vi "Unit_Test_Driver.vi"() -> ()   [LabVIEW 2019]
uses:
  <userlib>/LevyLab/Relay Box/Typedefs/Resistor--enum.ctl
  <userlib>/LevyLab/Relay Box/Relay-Box.lvclass
  lvsrc/subVIs/AFM API/AFM_Driver_Manager/AFM_Driver_Manager.PublicMethods.ctl
  lvsrc/subVIs/AFM API/AFM_Driver_Manager/AFM_Driver_Manager.lvclass
  lvsrc/subVIs/AFM API/AFM_Driver_Manager/AFM_Driver_Manager.PublicEvents.ctl
  <vilib>/addons/_JKI Toolkits/Caraya/classes/Test/Test.lvclass
  <vilib>/addons/_JKI Toolkits/Caraya/classes/Assert/Assert.lvclass
  <vilib>/addons/_JKI Toolkits/Caraya/classes/Assert/Assert True.vi
  <vilib>/addons/_JKI Toolkits/Caraya/classes/Assert/Assert Equal Value_Variant.vi
  <vilib>/addons/_JKI Toolkits/Caraya/classes/Assert/Assert False.vi
panel:
  in  "Levylab_Public_Events_Do_Not_Rename":T1
  in  "Levylab_Public_Methods_Do_Not_Rename":T2
  # "AFM Driver Template"
  # "UNIT TESTS"
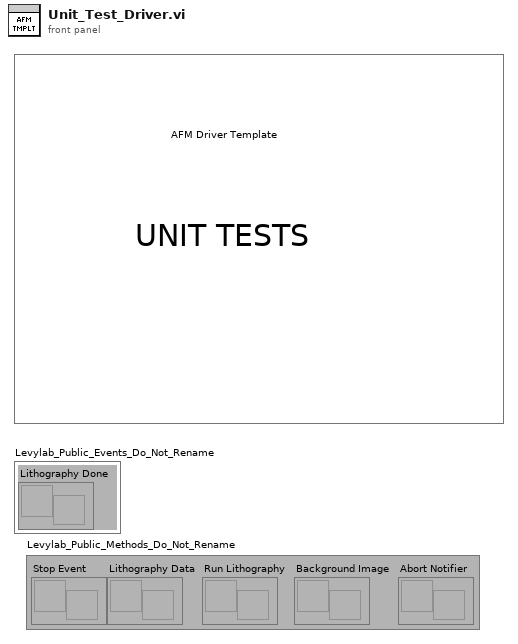
[diagram p1: front panel]
types:
  T1 = typedef "AFM_Driver_Manager.lvclass/AFM_Driver_Manager.PublicEvents.ctl" = cluster{"Lithography Done":refnum<user-event>}
  T2 = typedef "AFM_Driver_Manager.lvclass/AFM_Driver_Manager.PublicMethods.ctl" = cluster{"Stop Event":refnum<user-event>, "Lithography Data":refnum<user-event>, "Run Lithography":refnum<user-event>, "Background Image":refnum<user-event>, "Abort Notifier":refnum<user-event>}
  T3 = typedef "Relay-Box.lvclass/Resistor--enum.ctl" = enum16{"open", "discharge tip", "0 ohms", "100k ohm", "10M ohm", "1G ohm"}
  T4 = cluster{"Name":string, "Litho":cluster{"X":dbl, "Y":dbl, "Speed":dbl, "Voltage":dbl}[], "Set Resistance":T3, "Meta":variant}[]
  T5 = enum32{"Invalid", "Standard", "Closed", "Hidden", "Minimized", "Maximized"}
  T6 = enum32{"invalid app kind", "Development System", "Run Time System", "Student Edition", "Embedded LabVIEW", "Evaluation", "Custom"}
  T7 = cluster{"Core":cluster{"Current VI Reference":refnum<vi>, "Close Panel on Exit?":bool}, "Events":T1, "Lithography Data":cluster{"Name":string, "Litho":cluster{"X":dbl, "Y":dbl, "Speed":dbl, "Voltage":dbl}[], "Set Resistance":T3, "Meta":variant}[], "Background Image":path, "Abort Notifier":refnum<notifier>, "Offsets":cluster{"X":dbl, "Y":dbl}}
  T8 = cluster{"Current VI Reference":refnum<vi>, "Close Panel on Exit?":bool}
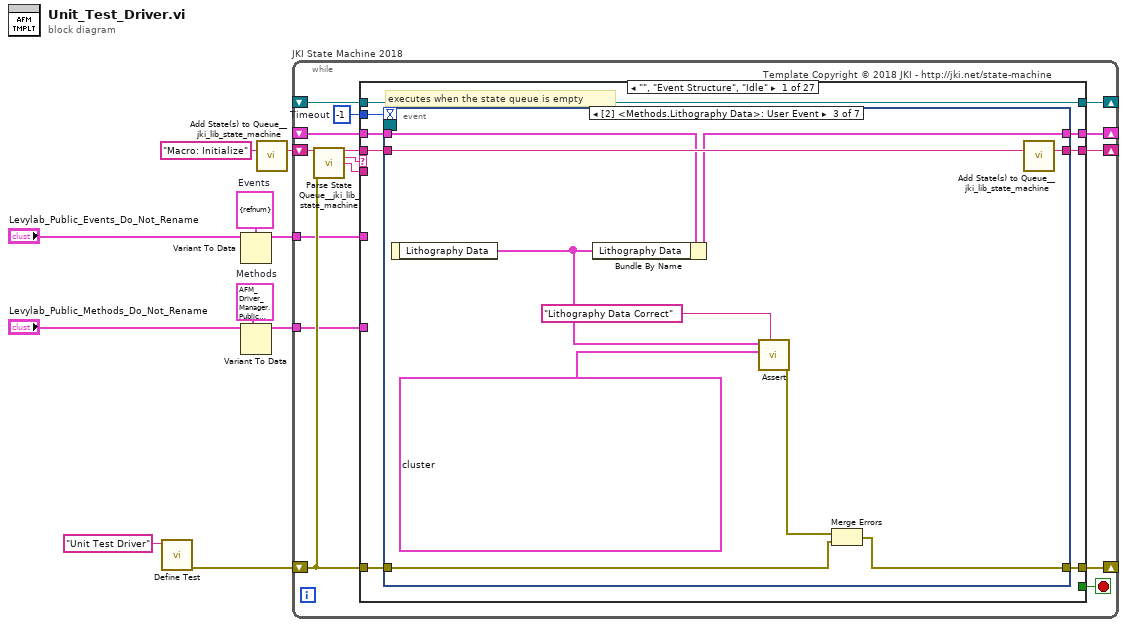
[diagram p0: block diagram]
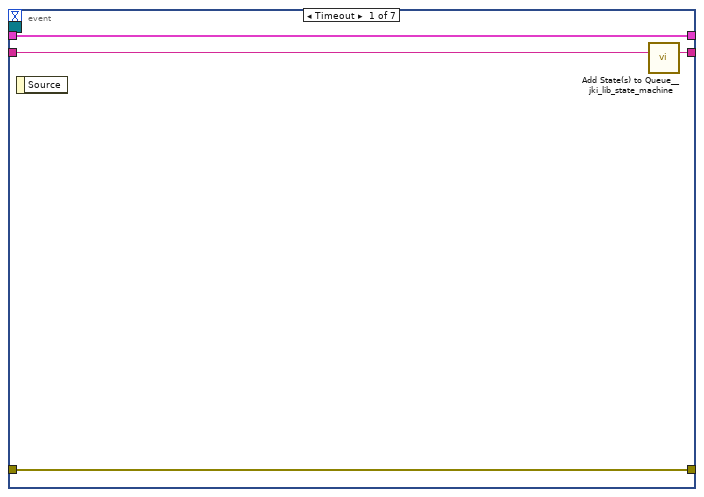
[diagram p2: hidden frame]
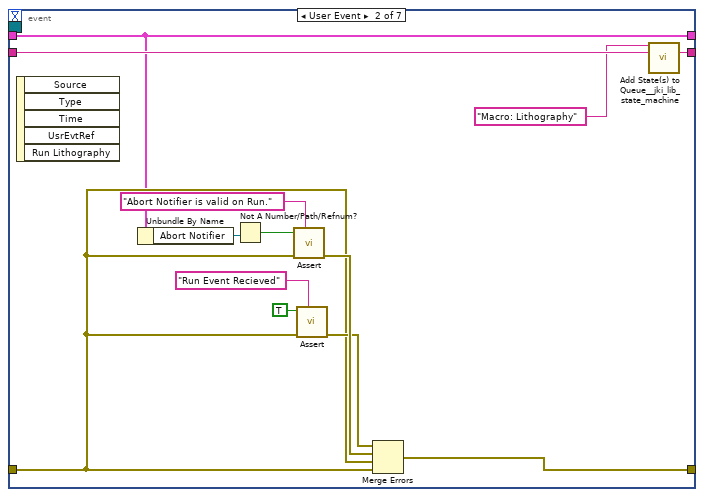
[diagram p3: hidden frame]
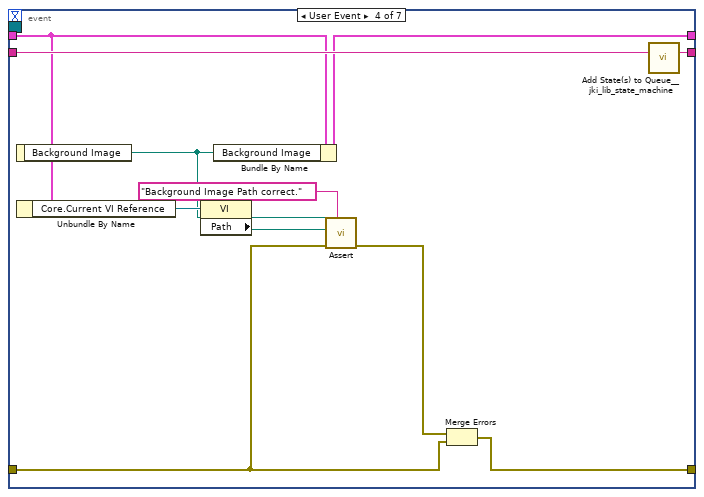
[diagram p4: hidden frame]
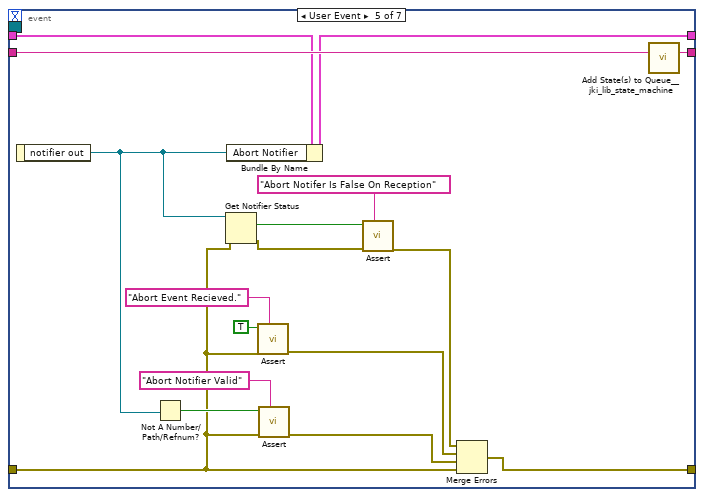
[diagram p5: hidden frame]
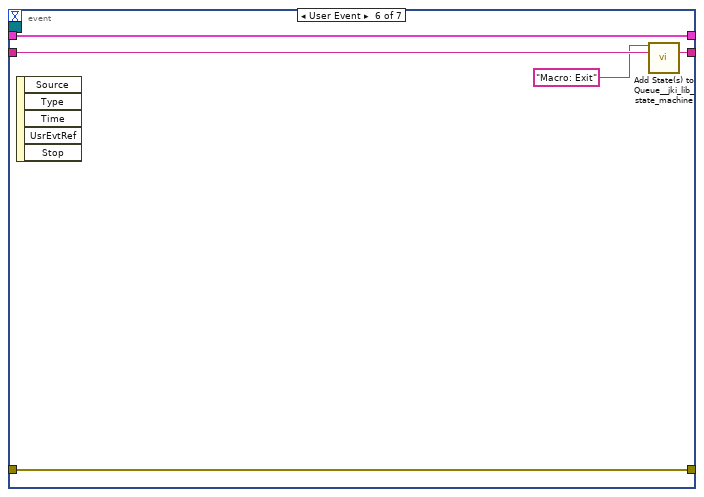
[diagram p6: hidden frame]
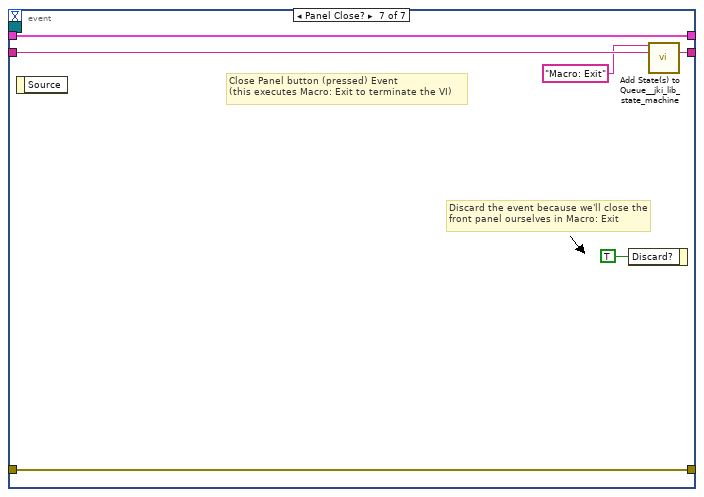
[diagram p7: hidden frame]
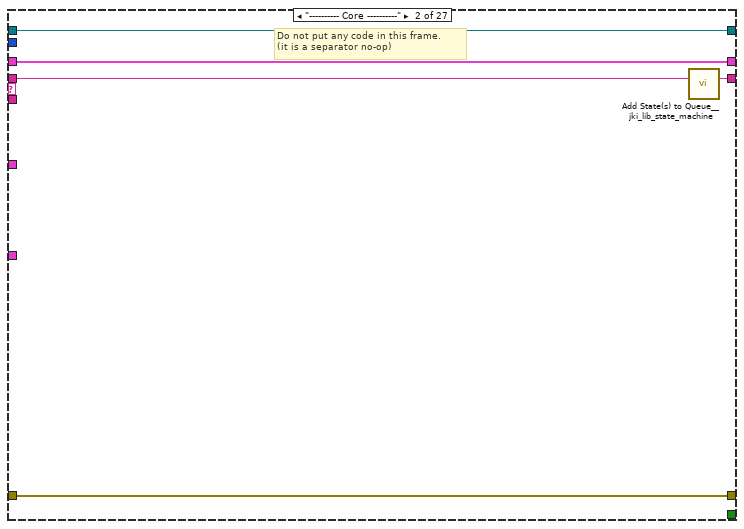
[diagram p8: hidden frame]
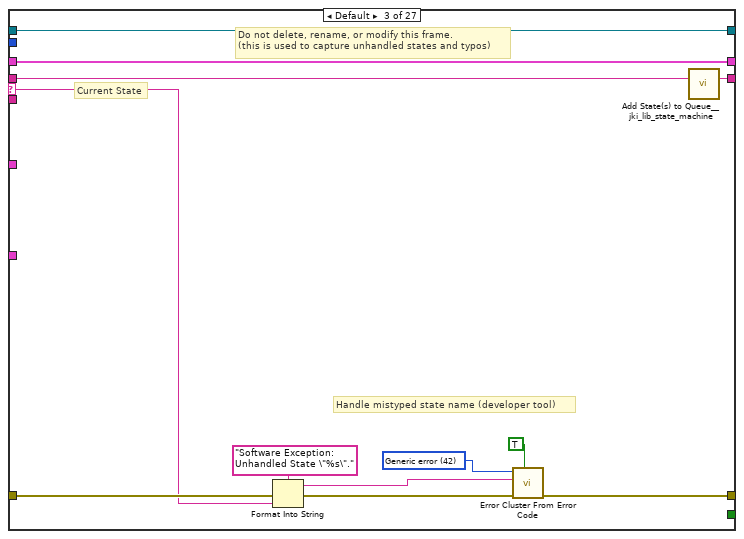
[diagram p9: hidden frame]
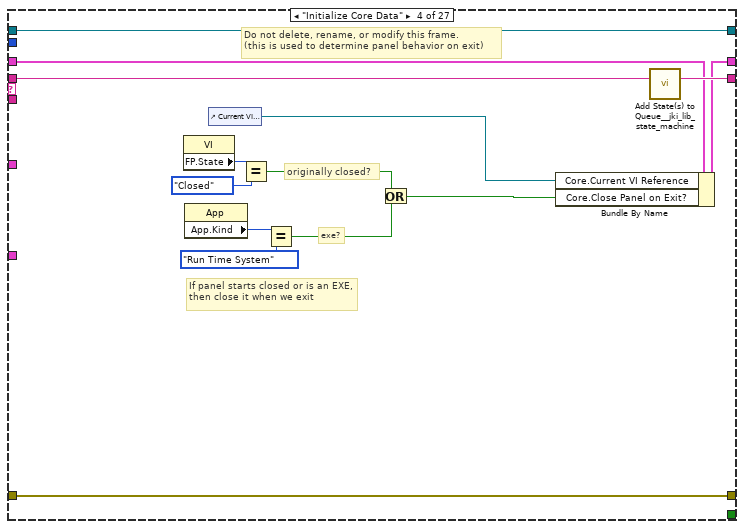
[diagram p10: hidden frame]
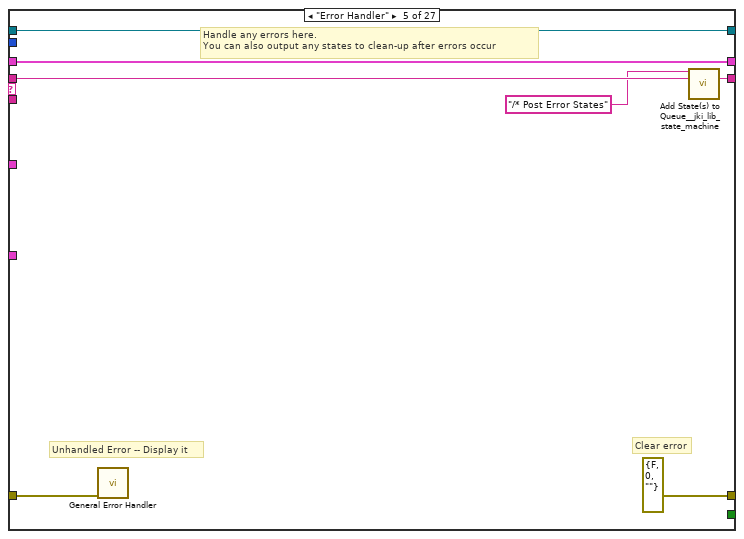
[diagram p11: hidden frame]
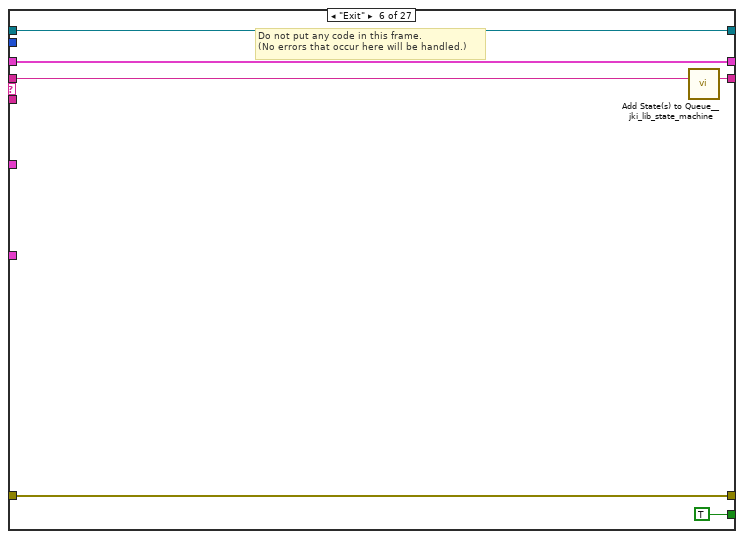
[diagram p12: hidden frame]
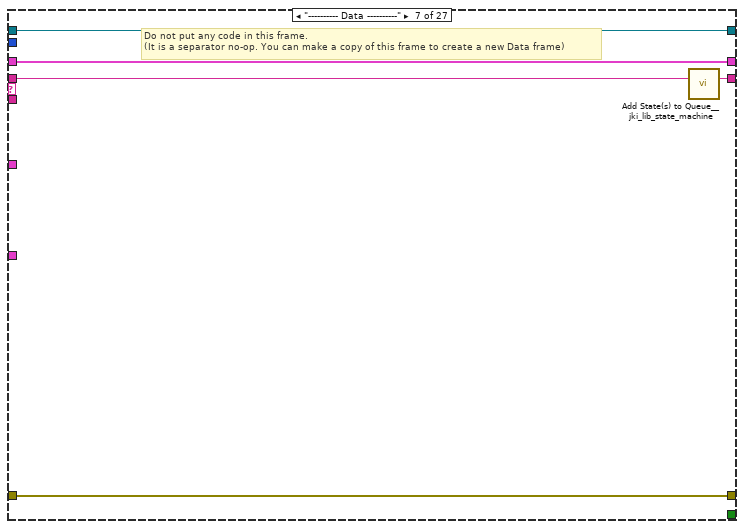
[diagram p13: hidden frame]
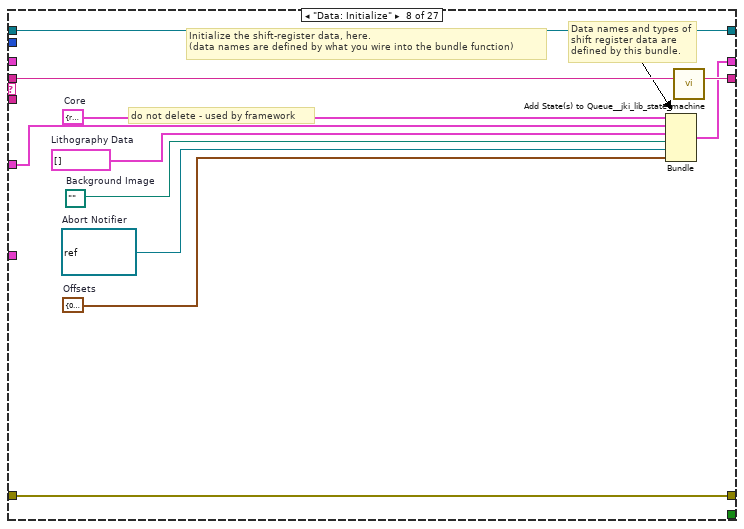
[diagram p14: hidden frame]
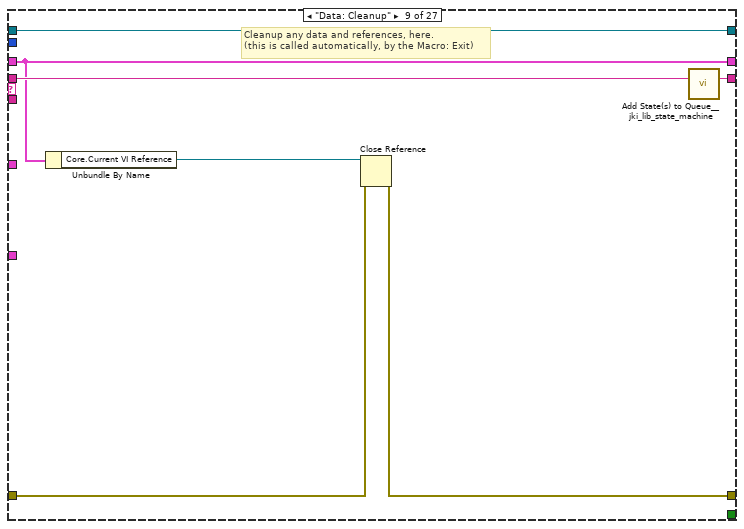
[diagram p15: hidden frame]
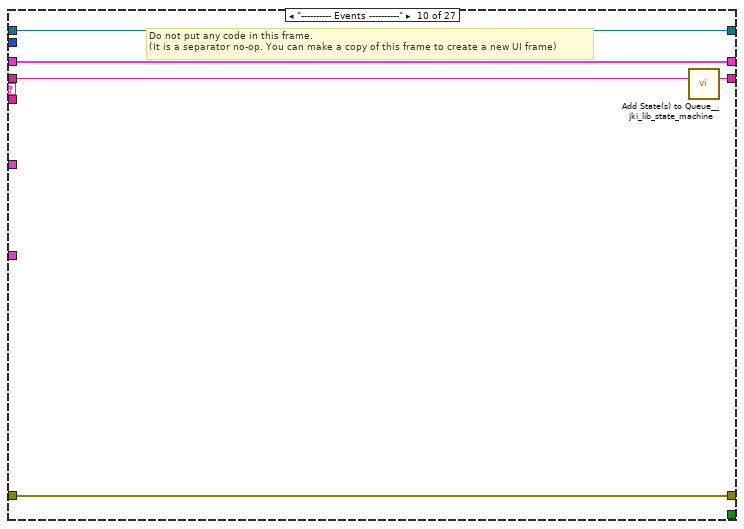
[diagram p16: hidden frame]
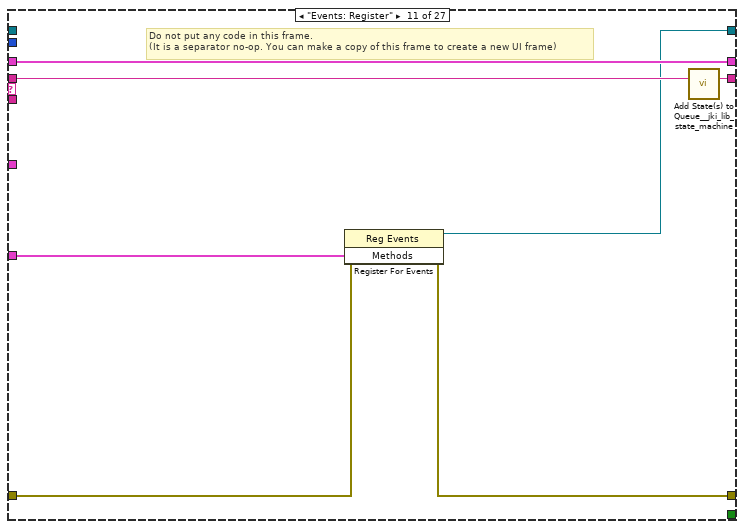
[diagram p17: hidden frame]
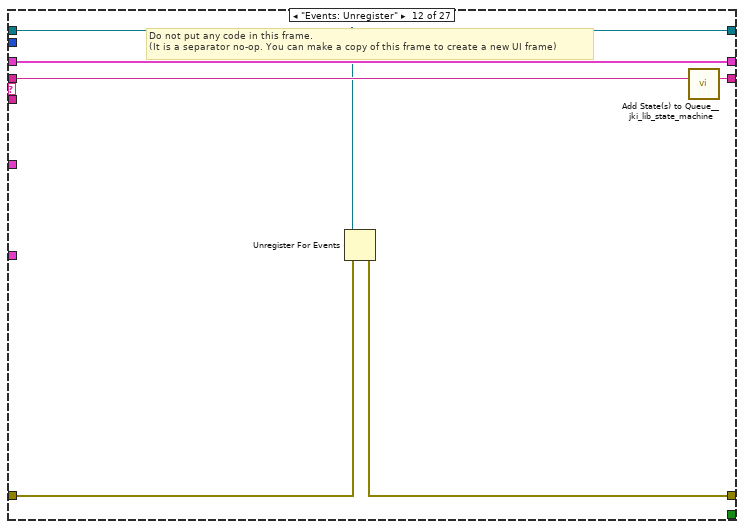
[diagram p18: hidden frame]
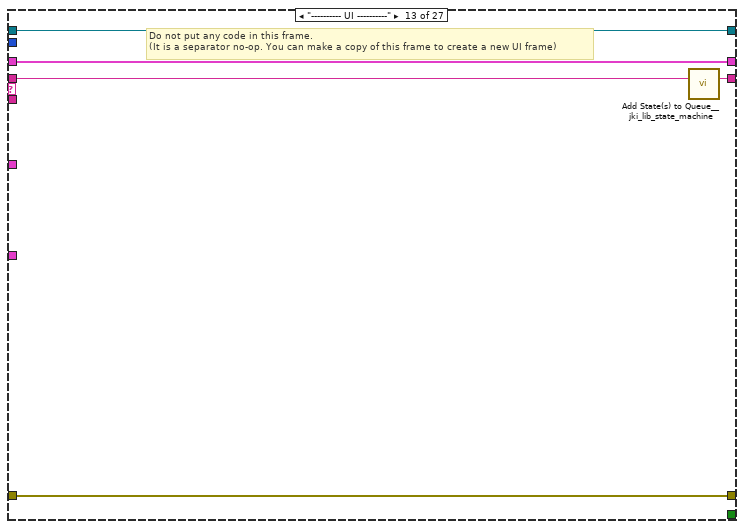
[diagram p19: hidden frame]
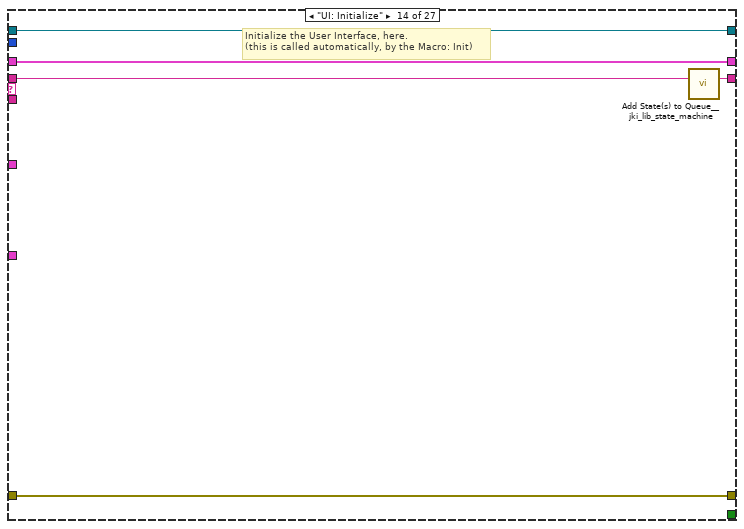
[diagram p20: hidden frame]
diagram:
  w6 = T1 {"Lithography Done"=refnum}  # Events
  w8 = T2 {"Stop Event"=refnum, "Lithography Data"=refnum, "Run Lithography"=refnum, "Background Image"=refnum, "Abort Notifier"=refnum}  # Methods
  n1 = call <vilib>:"Define Test.vi"("Label (VI Title)"="Unit Test Driver") -> ("error out"=w2:errorcluster)  [unwired: 9 in, 1 out]
  n2 = Variant To Data(type=w6, Variant="Levylab_Public_Events_Do_Not_Rename") -> (data=w3:T1)  [unwired: 1 in, 1 out]
  n3 = Variant To Data(type=w8, Variant="Levylab_Public_Methods_Do_Not_Rename") -> (data=w4:T2)  [unwired: 1 in, 1 out]
  n4 = call <vilib>:"Add State(s) to Queue__jki_lib_state_machine.vi"("State(s) in (\"\")"="Macro: Initialize") -> ("States Out"=w10:string)  [unwired: 14 in]
  n5 = while "JKI State Machine 2018" {
    shift-right: [w18] -> _
    shift-left: _ -> [w17]
    shift-right: [w21] -> _
    shift-left: w2 -> [w15]
    shift-right: [w20] -> _
    shift-left: w10 -> [w22]
    tunnel: w4 -> [w11]
    tunnel: w3 -> [w14]
    shift-right: [w13] -> _
    shift-left: _ -> [w12]
    stop <- w19 stop-if-true
    w16 = -1  # Timeout
    # "Template Copyright © 2018 JKI - http://jki.net/state-machine"
    n6 = call <vilib>:"Parse State Queue__jki_lib_state_machine.vi"("State Queue"=w22, "Error In (no error)"=w15) -> ("Remaining States"=w24:string, "Current State"=w25:string, "Arguments"=w23:string)  [unwired: 11 in]
    n7 = case shown="\"\", \"Event Structure\", \"Idle\"" w25 {
      selector: w25 -> [_ _ w106 _ _ _ _ _ _ _ _ _ _ _ _ _ _ _ _ _ _ _ _ _ _ _ _]
      tunnel: w24 -> [w33 w104 w110 w130 w137 w143 w148 w159 w166 w171 w178 w184 w189 w194 w201 w213 w283 w289 w295 w306 w311 w316 w321 w326 w331 w342 w358]
      tunnel: w23 -> [_ _ _ _ _ _ _ _ _ _ _ _ _ _ w196 w207 _ _ _ _ _ _ _ _ _ _ _]
      tunnel: w17 -> [w31 w101 w108 w123 w134 w141 w145 _ w161 w168 w176 w182 w186 w192 w199 w209 w280 w286 w292 w303 w308 w313 w318 w323 w328 w339 w355]
      tunnel: [w30 w102 w112 w127 errorcluster {"status"=FALSE, "code"=0, "source"=""} ("error out") w140 w146 w156 w162 w169 w172 w179 w187 w191 w197 w210 w281 w287 w293 w304 w309 w314 w319 w324 w329 w334 w352] -> w21
      tunnel: w15 -> [w29 w102 w111 w127 w133 w140 w146 w156 w163 w169 w173 w180 w187 w191 w198 w211 w281 w287 w293 w304 w309 w314 w319 w324 w329 w333 w351]
      tunnel: [w32 w103 w109 w129 w136 w142 w147 w158 w165 w170 w177 w183 w188 w193 w200 w212 w282 w288 w294 w305 w310 w315 w320 w325 w330 w341 w357] -> w20
      tunnel: [_ _ _ _ _ TRUE _ _ _ _ _ _ _ _ _ _ _ _ _ _ _ _ _ _ _ _ _] -> w19
      tunnel: [w28 w101 w108 w128 w134 w141 w145 w157 w161 w168 w176 w182 w186 w192 w199 w209 w280 w286 w292 w303 w308 w313 w318 w323 w328 w339 w355] -> w18
      tunnel: w16 -> [w27 _ _ _ _ _ _ _ _ _ _ _ _ _ _ _ _ _ _ _ _ _ _ _ _ _ _]
      tunnel: w14 -> [_ _ _ _ _ _ _ w154 _ _ _ _ _ _ _ _ _ _ _ _ _ _ _ _ _ _ _]
      tunnel: [w26 w100 w105 w117 w131 w138 w144 w150 w160 w167 w175 w181 w185 w190 w195 w206 w279 w284 w291 w296 w307 w312 w317 w322 w327 w340 w356] -> w13
      tunnel: w12 -> [w26 w100 w105 w117 w131 w138 w144 w150 w160 w167 _ w181 w185 w190 w195 w206 w279 w284 w291 w296 w307 w312 w317 w322 w327 w340 w356]
      tunnel: w11 -> [_ _ _ _ _ _ _ _ _ _ w174 _ _ _ _ _ _ _ _ _ _ _ _ _ _ _ _]
      frame "", "Event Structure", "Idle" {
        # "executes when the state queue is empty"
        n8 = event shown="[2] <Methods.Lithography Data>: User Event" {
          selector: w26 -> [_ _ _ _ _ _ _]
          dyn-events: _ -> [_ _ _ _ _ _ _]
          timeout: w27 -> [_ _ _ _ _ _ _]
          tunnel: w33 -> [w37 w50 w60 w71 w88 w93 w99]
          tunnel: [w36 w49 w59 w70 w87 w92 w98] -> w32
          tunnel: w31 -> [w34 w39 w57 w68 w85 w90 w96]
          tunnel: [w35 w43 w53 w63 w80 w91 w97] -> w30
          tunnel: w29 -> [w35 w40 w52 w61 w75 w91 w97]
          tunnel: [w34 w39 w58 w69 w86 w90 w96] -> w28
          event Timeout {
            n9 = event-data() -> ()  [unwired: 1 in, 1 out]
            n10 = call <vilib>:"Add State(s) to Queue__jki_lib_state_machine.vi"("State(s) in (\"\")"=w37) -> ("States Out"=w36:string)  [unwired: 14 in]
          }
          event User Event {
            n11 = event-data() -> ()  [unwired: 1 in, 5 out]
            n12 = Unbundle By Name(w39) -> ("Abort Notifier"=w38:refnum<notifier>)
            n13 = Not A Number/Path/Refnum?(number/path/refnum=w38) -> (NaN/Path/Refnum?=w46:bool)
            n14 = call-poly <vilib>:"Assert.vi"("Label"="Abort Notifier is valid on Run.", "error in (no error)"=w40, "False?"=w46) -> ("error out"=w42:errorcluster)  [unwired: 7 in, 1 out]
            n15 = call-poly <vilib>:"Assert.vi"("Label"="Run Event Recieved", "error in (no error)"=w40, "True?"=TRUE) -> ("error out"=w41:errorcluster)  [unwired: 7 in, 1 out]
            n16 = Merge Errors(w41, w42, w40, w40) -> (w43:errorcluster)
            n17 = call <vilib>:"Add State(s) to Queue__jki_lib_state_machine.vi"("State(s) in Front (\"\")"="Macro: Lithography", "State(s) in (\"\")"=w50) -> ("States Out"=w49:string)  [unwired: 13 in]
          }
          event User Event {
            n18 = event-data() -> ("Lithography Data"=w51:T4)  [unwired: 1 in]
            n19 = Bundle By Name(cluster=w57, "Lithography Data"=w51) -> (w58:T7)
            n20 = call-poly <vilib>:"Assert.vi"("Label"="Lithography Data Correct", "Y"=T4 [{"Name"="p0", "Litho"=[{"X"=1.0, "Y"=2.0, "Speed"=3.0, "Voltage"=4.0}], "Set Resistance"=enum."discharge tip", "Meta"=variant}, {"Name"="p1", "Litho"=[{"X"=5.0, "Y"=6.0, "Speed"=7.0, "Voltage"=8.0}], "Set Resistance"=enum."open", "Meta"=variant}] ("Lithography Data"), "X"=w51) -> ("error out"=w54:errorcluster)  [unwired: 7 in, 1 out]
            n21 = Merge Errors(w54, w52) -> (w53:errorcluster)
            n22 = call <vilib>:"Add State(s) to Queue__jki_lib_state_machine.vi"("State(s) in (\"\")"=w60) -> ("States Out"=w59:string)  [unwired: 14 in]
          }
          event User Event {
            n23 = event-data() -> ("Background Image"=w66:path)  [unwired: 1 in]
            n24 = Unbundle By Name(w68) -> ("Core.Current VI Reference"=w67:refnum<vi>)
            n25 = property class="VI"(reference=w67) -> ("Path"=w65:path)  [unwired: 1 in, 2 out]
            n26 = Bundle By Name(cluster=w68, "Background Image"=w66) -> (w69:T7)
            n27 = call-poly <vilib>:"Assert.vi"("Label"="Background Image Path correct.", "error in (no error)"=w61, "Y"=w65, "X"=w66) -> ("error out"=w62:errorcluster)  [unwired: 6 in, 1 out]
            n28 = Merge Errors(w62, w61) -> (w63:errorcluster)
            n29 = call <vilib>:"Add State(s) to Queue__jki_lib_state_machine.vi"("State(s) in (\"\")"=w71) -> ("States Out"=w70:string)  [unwired: 14 in]
          }
          event User Event {
            n30 = event-data() -> ("notifier out"=w74:refnum<notifier>)  [unwired: 1 in]
            n31 = Not A Number/Path/Refnum?(number/path/refnum=w74) -> (NaN/Path/Refnum?=w82:bool)
            n32 = Get Notifier Status(notifier=w74, error in (no error)=w75) -> (current notification=w73:bool, error out=w76:errorcluster)  [unwired: 3 out]
            n33 = Bundle By Name(cluster=w85, "Abort Notifier"=w74) -> (w86:T7)
            n34 = call-poly <vilib>:"Assert.vi"("Label"="Abort Event Recieved.", "error in (no error)"=w75, "True?"=TRUE) -> ("error out"=w79:errorcluster)  [unwired: 7 in, 1 out]
            n35 = call-poly <vilib>:"Assert.vi"("Label"="Abort Notifier Valid", "error in (no error)"=w75, "False?"=w82) -> ("error out"=w78:errorcluster)  [unwired: 7 in, 1 out]
            n36 = call-poly <vilib>:"Assert.vi"("Label"="Abort Notifer Is False On Reception", "error in (no error)"=w76, "False?"=w73) -> ("error out"=w77:errorcluster)  [unwired: 7 in, 1 out]
            n37 = Merge Errors(w77, w79, w78, w75) -> (w80:errorcluster)
            n38 = call <vilib>:"Add State(s) to Queue__jki_lib_state_machine.vi"("State(s) in (\"\")"=w88) -> ("States Out"=w87:string)  [unwired: 14 in]
          }
          event User Event {
            n39 = event-data() -> ()  [unwired: 1 in, 5 out]
            n40 = call <vilib>:"Add State(s) to Queue__jki_lib_state_machine.vi"("State(s) in Front (\"\")"="Macro: Exit", "State(s) in (\"\")"=w93) -> ("States Out"=w92:string)  [unwired: 13 in]
          }
          event Panel Close? {
            # "Discard the event because we'll close the front panel ourselves in Macro: Exit"
            # "Close Panel button (pressed) Event\n(this executes Macro: Exit to terminate the VI)"
            n41 = event-data() -> ()  [unwired: 1 in, 1 out]
            n42 = event-data("Discard?"=TRUE) -> ()  [unwired: 1 in, 1 out]
            n43 = call <vilib>:"Add State(s) to Queue__jki_lib_state_machine.vi"("State(s) in Front (\"\")"="Macro: Exit", "State(s) in (\"\")"=w99) -> ("States Out"=w98:string)  [unwired: 13 in]
          }
        }
      }
      frame "---------- Core ----------" {
        # "Do not put any code in this frame.\n(it is a separator no-op)"
        n44 = call <vilib>:"Add State(s) to Queue__jki_lib_state_machine.vi"("State(s) in (\"\")"=w104) -> ("States Out"=w103:string)  [unwired: 14 in]
      }
      frame Default {
        w115 = 42 items=["No error", "Argument error", "Memory is full", "Out of zone", "End of file", "File already open", "Generic file I/O error", "File not found", "File permission error", "Disk is full", "Duplicate path", "Too many files open", "System feature not enabled", "Resource file not found", "Cannot add resource", "Resource not found", "Image not found", "Image memory error", "Pen does not exist", "Config type invalid", "Config token not found", "Config parse error", "Config memory error", "Bad external code format", "Bad external code offset", "External code not present", "Null window", "Destroy window error", "Null menu", "Print aborted", "Bad print record", "Print driver error", "Windows error during printing", "Memory error during printing", "Print dialog error", "Generic print error", "Invalid device refnum", "Device not found", "Device parameter error", "Device unit error", "Cannot open device", "Device call aborted", "Generic error", "Cancelled by user", "Object ID too low", "Object ID too high", "Object not in heap", "Unknown heap", "Unknown object (invalid DefProc)", "Unknown object (DefProc not in table)", "Message out of range", "Invalid (null) method", "Unknown message", "Manager call not supported", "Bad address", "Network operation in progress", "Network operation timed out", "Connection is busy", "Network attribute not supported", "Network error", "Address in use", "System out of memory", "Connection aborted", "Connection refused", "Not connected", "Already connected", "Connection closed", "Initialization error (interapplication manager)", "Bad occurrence", "Wait on unbound occurrence handler", "Occurrence queue overflow", "Datalog type conflict", "Unused", "Unrecognized type (interapplication manager)", "Memory corrupt", "Failed to make temporary DLL", "Old CIN version", "Drag socket not found", "Failed to load drop-object", "Failed to register OLE object", "Failed to release OLE object", "Format specifier type mismatch", "Unknown format specifier", "Too few format specifiers", "Too many format specifiers", "Scan failed", "Newer CIN version", "Error converting to variant", "Runtime menu error", "Password tampered", "Variant attribute not found", "Incompatible variant data type", "Event data is not available", "Event Store is not present", "Occurrence is not found", "Event Queue is not created", "Event info is not available", "Refnum passed is NULL", "Error retrieving Class GUID", "Error retrieving CoClass GUID", "Error retrieving TypeLib GUID.", "Bad built application magic bytes.", "Specific driver is different from the specific driver associated with the Logical Name.", "There is no session opened to the class driver.", "Max Error", "MAX - Error with config objects", "MAX - Error loading configuration", "MAX - Group not supported"]
        # "Current State"
        # "Do not delete, rename, or modify this frame.\n(this is used to capture unhandled states and typos)"
        # "Handle mistyped state name (developer tool)"
        n45 = Format Into String(format string="Software Exception: Unhandled State \"%s\"." ("message"), error in=w111, w106) -> (resulting string=w114:string, error out=w113:errorcluster)  [unwired: 1 in]
        n46 = call <vilib>:"Error Cluster From Error Code.vi"("show call chain? (False)"=TRUE, "error in (no error)"=w113, "error message (\"\")"=w114, "error code (0)"=w115) -> ("error out"=w112:errorcluster)  [unwired: 5 in]
        n47 = call <vilib>:"Add State(s) to Queue__jki_lib_state_machine.vi"("State(s) in (\"\")"=w110) -> ("States Out"=w109:string)  [unwired: 14 in]
      }
      frame "Initialize Core Data" {
        # "Do not delete, rename, or modify this frame.\n(this is used to determine panel behavior on exit)"
        # "originally closed?"
        # "exe?"
        # "If panel starts closed or is an EXE, then close it when we exit"
        n48 = property class="VI"() -> ("FP.State"=w120:T5)  [unwired: 2 in, 2 out]
        n49 = property class="App"() -> ("App.Kind"=w126:T6)  [unwired: 2 in, 2 out]
        n50 = control-ref of="Current VI Reference"() -> (w121:refnum<vi>)
        n51 = Equal?(x=w120, y=T5."Closed" ("Front Panel Window:State")) -> (x = y?=w118:bool)
        n52 = Equal?(x=w126, y=T6."Run Time System" ("Application:Kind")) -> (x = y?=w124:bool)
        n53 = Or(x=w118, y=w124) -> (x .or. y?=w122:bool)
        n54 = Bundle By Name(cluster=w123, "Core.Current VI Reference"=w121, "Core.Close Panel on Exit?"=w122) -> (w128:T7)
        n55 = call <vilib>:"Add State(s) to Queue__jki_lib_state_machine.vi"("State(s) in (\"\")"=w130) -> ("States Out"=w129:string)  [unwired: 14 in]
      }
      frame "Error Handler" {
        # "Unhandled Error -- Display it"
        # "Handle any errors here.\nYou can also output any states to clean-up after errors occur"
        # "Clear error"
        n56 = call <vilib>:"General Error Handler.vi"("error in (no error)"=w133) -> ()  [unwired: 10 in, 5 out]
        n57 = call <vilib>:"Add State(s) to Queue__jki_lib_state_machine.vi"("State(s) in Front (\"\")"="/* Post Error States", "State(s) in (\"\")"=w137) -> ("States Out"=w136:string)  [unwired: 13 in]
      }
      frame "Exit" {
        # "Do not put any code in this frame.\n(No errors that occur here will be handled.)"
        n58 = call <vilib>:"Add State(s) to Queue__jki_lib_state_machine.vi"("State(s) in (\"\")"=w143) -> ("States Out"=w142:string)  [unwired: 14 in]
      }
      frame "---------- Data ----------" {
        # "Do not put any code in this frame.\n(It is a separator no-op. You can make a copy of this frame to create a new Data frame)"
        n59 = call <vilib>:"Add State(s) to Queue__jki_lib_state_machine.vi"("State(s) in (\"\")"=w148) -> ("States Out"=w147:string)  [unwired: 14 in]
      }
      frame "Data: Initialize" {
        w149 = T4 []  # Lithography Data
        w152 = refnum<notifier> refnum  # Abort Notifier
        w151 = cluster{"X":dbl, "Y":dbl} {"X"=0.0, "Y"=0.0}  # Offsets
        w153 = path ""  # Background Image
        w155 = T8 {"Current VI Reference"=refnum, "Close Panel on Exit?"=FALSE}  # Core
        # "do not delete - used by framework"
        # "Data names and types of shift register data are defined by this bundle."
        # "Initialize the shift-register data, here.\n(data names are defined by what you wire into the bundle function)"
        n60 = Bundle("Core"=w155, "Events"=w154, "Lithography Data"=w149, "Background Image"=w153, "Abort Notifier"=w152, "Offsets"=w151) -> (w157:T7)  [unwired: 1 in]
        n61 = call <vilib>:"Add State(s) to Queue__jki_lib_state_machine.vi"("State(s) in (\"\")"=w159) -> ("States Out"=w158:string)  [unwired: 14 in]
      }
      frame "Data: Cleanup" {
        # "Cleanup any data and references, here.\n(this is called automatically, by the Macro: Exit)"
        n62 = Unbundle By Name(w161) -> ("Core.Current VI Reference"=w164:refnum<vi>)
        n63 = Close Reference(reference=w164, error in (no error)=w163) -> (error out=w162:errorcluster)
        n64 = call <vilib>:"Add State(s) to Queue__jki_lib_state_machine.vi"("State(s) in (\"\")"=w166) -> ("States Out"=w165:string)  [unwired: 14 in]
      }
      frame "---------- Events ----------" {
        # "Do not put any code in this frame.\n(It is a separator no-op. You can make a copy of this frame to create a new UI frame)"
        n65 = call <vilib>:"Add State(s) to Queue__jki_lib_state_machine.vi"("State(s) in (\"\")"=w171) -> ("States Out"=w170:string)  [unwired: 14 in]
      }
      frame "Events: Register" {
        # "Do not put any code in this frame.\n(It is a separator no-op. You can make a copy of this frame to create a new UI frame)"
        n66 = register-events(error in=w173, w174) -> (reference out=w175:refnum<event-registration>, error out=w172:errorcluster)  [unwired: 1 in]
        n67 = call <vilib>:"Add State(s) to Queue__jki_lib_state_machine.vi"("State(s) in (\"\")"=w178) -> ("States Out"=w177:string)  [unwired: 14 in]
      }
      frame "Events: Unregister" {
        # "Do not put any code in this frame.\n(It is a separator no-op. You can make a copy of this frame to create a new UI frame)"
        n68 = Unregister For Events(event registration refnum=w181, error in=w180) -> (error out=w179:errorcluster)
        n69 = call <vilib>:"Add State(s) to Queue__jki_lib_state_machine.vi"("State(s) in (\"\")"=w184) -> ("States Out"=w183:string)  [unwired: 14 in]
      }
      frame "---------- UI ----------" {
        # "Do not put any code in this frame.\n(It is a separator no-op. You can make a copy of this frame to create a new UI frame)"
        n70 = call <vilib>:"Add State(s) to Queue__jki_lib_state_machine.vi"("State(s) in (\"\")"=w189) -> ("States Out"=w188:string)  [unwired: 14 in]
      }
      frame "UI: Initialize" {
        # "Initialize the User Interface, here.\n(this is called automatically, by the Macro: Init)"
        n71 = call <vilib>:"Add State(s) to Queue__jki_lib_state_machine.vi"("State(s) in (\"\")"=w194) -> ("States Out"=w193:string)  [unwired: 14 in]
      }
      frame "UI: Cursor Set" {
        # "Argument"
        # "Set and Unset Cursor Busy.\n(Usage: \"UI: Cursor Set >> Busy|Idle\")"
        n72 = case shown="\"Idle\", Default" w196 {
          tunnel: w198 -> [w203 w205]
          tunnel: [w202 w204] -> w197
          frame "Idle", Default {
            n73 = call <vilib>:"Unset Busy.vi"("error in (no error)"=w203) -> ("error out"=w202:errorcluster)  [unwired: 10 in]
          }
          frame "Busy" {
            n74 = call <vilib>:"Set Busy.vi"("error in (no error)"=w205) -> ("error out"=w204:errorcluster)  [unwired: 9 in, 1 out]
          }
        }
        n75 = call <vilib>:"Add State(s) to Queue__jki_lib_state_machine.vi"("State(s) in (\"\")"=w201) -> ("States Out"=w200:string)  [unwired: 14 in]
      }
      frame "UI: Front Panel State" {
        # "Argument"
        # "Set Front Panel Open or Closed\n(Usage: \"UI: Front Panel State >> Open|Close\")"
        n76 = Unbundle By Name(w209) -> ("Core.Current VI Reference"=w208:refnum<vi>)
        n77 = case shown="\"Minimize\", \"Minimized\"" w207 {
          tunnel: w211 -> [w219 w234 w245 w258 w271]
          tunnel: [w221 w235 w247 w260 w273] -> w210
          tunnel: w208 -> [w220 w232 w246 w259 w272]
          frame "Open", "Standard", Default {
            w214 = T5."Standard" ("State")
            n78 = property class="VI"(reference=w220, error in=w219) -> (reference out=w217:refnum<vi>, error out=w218:errorcluster, "FP.State"=w216:T5)
            n79 = Not Equal?(x=w216, y=w214) -> (x != y?=w215:bool)
            n80 = case shown="True" w215 {
              tunnel: [w225 w227] -> w221
              tunnel: w218 -> [w224 w227]
              tunnel: w217 -> [w223 _]
              tunnel: w214 -> [w222 _]
              frame True {
                n81 = invoke class="VI" method="FP.Open"(reference=w223, error in=w224, "Activate"=TRUE, "State"=w222) -> (error out=w225:errorcluster)  [unwired: 1 in, 4 out]
              }
              frame False {
              }
            }
          }
          frame "Close", "Closed" {
            n82 = property class="VI"(reference=w232, error in=w234) -> (reference out=w231:refnum<vi>, error out=w233:errorcluster, "FP.State"=w229:T5)
            n83 = Not Equal?(x=w229, y=T5."Closed" ("Front Panel Window:State")) -> (x != y?=w228:bool)
            n84 = case shown="True" w228 {
              tunnel: [w236 w239] -> w235
              tunnel: w233 -> [w236 w238]
              tunnel: w231 -> [_ w237]
              frame False {
              }
              frame True {
                n85 = invoke class="VI" method="FP.Close"(reference=w237, error in=w238) -> (error out=w239:errorcluster)  [unwired: 1 in, 2 out]
              }
            }
          }
          frame "Hidden", "Hide" {
            w240 = T5."Hidden" ("State")
            n86 = property class="VI"(reference=w246, error in=w245) -> (reference out=w243:refnum<vi>, error out=w244:errorcluster, "FP.State"=w242:T5)
            n87 = Not Equal?(x=w242, y=w240) -> (x != y?=w241:bool)
            n88 = case shown="True" w241 {
              tunnel: [w251 w252] -> w247
              tunnel: w244 -> [w250 w252]
              tunnel: w243 -> [w249 _]
              tunnel: w240 -> [w248 _]
              frame True {
                n89 = invoke class="VI" method="FP.Open"(reference=w249, error in=w250, "State"=w248) -> (error out=w251:errorcluster)  [unwired: 2 in, 4 out]
              }
              frame False {
              }
            }
          }
          frame "Minimize", "Minimized" {
            w253 = T5."Minimized" ("State")
            n90 = property class="VI"(reference=w259, error in=w258) -> (reference out=w256:refnum<vi>, error out=w257:errorcluster, "FP.State"=w255:T5)
            n91 = Not Equal?(x=w255, y=w253) -> (x != y?=w254:bool)
            n92 = case shown="True" w254 {
              tunnel: [w264 w265] -> w260
              tunnel: w257 -> [w263 w265]
              tunnel: w256 -> [w262 _]
              tunnel: w253 -> [w261 _]
              frame True {
                n93 = invoke class="VI" method="FP.Open"(reference=w262, error in=w263, "State"=w261) -> (error out=w264:errorcluster)  [unwired: 2 in, 4 out]
              }
              frame False {
              }
            }
          }
          frame "Maximize", "Maximized" {
            w266 = T5."Maximized" ("State")
            n94 = property class="VI"(reference=w272, error in=w271) -> (reference out=w269:refnum<vi>, error out=w270:errorcluster, "FP.State"=w268:T5)
            n95 = Not Equal?(x=w268, y=w266) -> (x != y?=w267:bool)
            n96 = case shown="True" w267 {
              tunnel: [w277 w278] -> w273
              tunnel: w270 -> [w276 w278]
              tunnel: w269 -> [w275 _]
              tunnel: w266 -> [w274 _]
              frame True {
                n97 = invoke class="VI" method="FP.Open"(reference=w275, error in=w276, "State"=w274) -> (error out=w277:errorcluster)  [unwired: 2 in, 4 out]
              }
              frame False {
              }
            }
          }
        }
        n98 = call <vilib>:"Add State(s) to Queue__jki_lib_state_machine.vi"("State(s) in (\"\")"=w213) -> ("States Out"=w212:string)  [unwired: 14 in]
      }
      frame "---------- Macro ----------" {
        # "Do not put any code in this frame.\n(It is a separator no-op. You can make a copy of this frame to create a new Macro frame)"
        n99 = call <vilib>:"Add State(s) to Queue__jki_lib_state_machine.vi"("State(s) in (\"\")"=w283) -> ("States Out"=w282:string)  [unwired: 14 in]
      }
      frame "Macro: Initialize" {
        # "Initialization Macro\n(This is called once, when the VI starts)"
        n100 = call <vilib>:"Add State(s) to Queue__jki_lib_state_machine.vi"("State(s) in Front (\"\")"="Data: Initialize\nInitialize Core Data\nEvents: Register\nUI: Initialize\n//UI: Front Panel State >> Open\nAFM: Open", "State(s) in (\"\")"=w289) -> ("States Out"=w288:string)  [unwired: 13 in]
      }
      frame "Macro: Lithography" {
        # "Do not put any code in this frame.\n(It is a separator no-op. You can make a copy of this frame to create a new Macro frame)"
        n101 = call <vilib>:"Add State(s) to Queue__jki_lib_state_machine.vi"("State(s) in Front (\"\")"="Lithography: Initialize\nLithography: Run\nLithography: Cleanup", "State(s) in (\"\")"=w295) -> ("States Out"=w294:string)  [unwired: 13 in]
      }
      frame "Macro: Exit" {
        # "Exit Macro\n(This is called once, when the VI exits)"
        n102 = Unbundle By Name(w303) -> ("Core.Close Panel on Exit?"=w302:bool)
        n103 = Select(t="UI: Front Panel State >> Close", s=w302, f="") -> (s? t:f=w299:string)
        n104 = call <vilib>:"Add State(s) to Queue__jki_lib_state_machine.vi"("State(s) in (\"\")"=w299, "State(s) at Back (\"\")"="AFM: Release\nData: Cleanup\nEvents: Unregister\nExit") -> ("States Out"=w297:string)  [unwired: 13 in]
        n105 = call <vilib>:"Add State(s) to Queue__jki_lib_state_machine.vi"("State(s) in Front (\"\")"=w297, "State(s) in (\"\")"=w306) -> ("States Out"=w305:string)  [unwired: 13 in]
      }
      frame "---------- AFM ----------" {
        # "Template Separator\n(You can make a copy of, or modify, this frame)"
        n106 = call <vilib>:"Add State(s) to Queue__jki_lib_state_machine.vi"("State(s) in (\"\")"=w311) -> ("States Out"=w310:string)  [unwired: 14 in]
      }
      frame "AFM: Release" {
        # "Close previously opened connection to the AFM Control Software Here\n(ActiveX, .NET, TCP, etc.)"
        n107 = call <vilib>:"Add State(s) to Queue__jki_lib_state_machine.vi"("State(s) in (\"\")"=w316) -> ("States Out"=w315:string)  [unwired: 14 in]
      }
      frame "AFM: Open" {
        # "Open a connection to the AFM Control Software Here\n(ActiveX, .NET, TCP, etc.)"
        n108 = call <vilib>:"Add State(s) to Queue__jki_lib_state_machine.vi"("State(s) in (\"\")"=w321) -> ("States Out"=w320:string)  [unwired: 14 in]
      }
      frame "---------- Lithography ----------" {
        # "Template Separator\n(You can make a copy of, or modify, this frame)"
        n109 = call <vilib>:"Add State(s) to Queue__jki_lib_state_machine.vi"("State(s) in (\"\")"=w326) -> ("States Out"=w325:string)  [unwired: 14 in]
      }
      frame "Lithography: Initialize" {
        # "Perform actions that need to happen before anything else:\n(Get Offsets, Perform scaling and translations, etc)"
        n110 = call <vilib>:"Add State(s) to Queue__jki_lib_state_machine.vi"("State(s) in (\"\")"=w331) -> ("States Out"=w330:string)  [unwired: 14 in]
      }
      frame "Lithography: Run" {
        # "Give 5 seconds for abort\n(should be called much sooner)"
        # "Perform the Lithography Sequence\n(Go through objects, moving to their initial points, setting tip down, running through all of the points in object etc.)"
        n111 = Unbundle By Name(w339) -> ("Abort Notifier"=w336:refnum<notifier>)
        n112 = Tick Count (ms)() -> (millisecond timer value=w338:u32)
        n113 = while {
          tunnel: w338 -> [w349]
          tunnel: u32 5000 -> [w348]
          tunnel: w336 -> [w346]
          tunnel: [w343] -> w335
          stop <- w344 stop-if-true
          n114 = Tick Count (ms)() -> (millisecond timer value=w350:u32)
          n115 = Subtract(x=w350, y=w349) -> (x-y=w347:u32)
          n116 = Get Notifier Status(notifier=w346) -> (current notification=w343:bool)  [unwired: 1 in, 4 out]
          n117 = Greater Or Equal?(x=w347, y=w348) -> (x >= y?=w345:bool)
          n118 = Or(x=w343, y=w345) -> (x .or. y?=w344:bool)
        }
        n119 = call-poly <vilib>:"Assert.vi"("Label"="Abort Called", "error in (no error)"=w333, "True?"=w335) -> ("error out"=w334:errorcluster)  [unwired: 7 in, 1 out]
        n120 = call <vilib>:"Add State(s) to Queue__jki_lib_state_machine.vi"("State(s) in (\"\")"=w342) -> ("States Out"=w341:string)  [unwired: 14 in]
      }
      frame "Lithography: Cleanup" {
        # "Perform any post lithography actions here + Tell world we are done with lithography\n(Make sure to send Lithography Done Event.)"
        n121 = Unbundle By Name(w355) -> ("Events.Lithography Done"=w354:refnum<user-event>)
        n122 = Generate User Event(user event=w354, event data cluster=TRUE ("event data"), error in=w351) -> (error out=w352:errorcluster)  [unwired: 1 in, 1 out]
        n123 = call <vilib>:"Add State(s) to Queue__jki_lib_state_machine.vi"("State(s) in (\"\")"=w358) -> ("States Out"=w357:string)  [unwired: 14 in]
      }
    }
  }
